vi "capex relay.vi"() -> ()   [LabVIEW 2013]
panel:
  in  "stop":bool
  in  "Relay 4":bool
  in  "Relay 3":bool
  in  "Relay 2":bool
  in  "Relay 1":bool
  # "Relays"
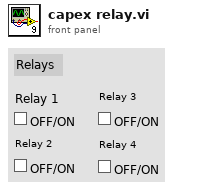
[diagram p1: front panel]
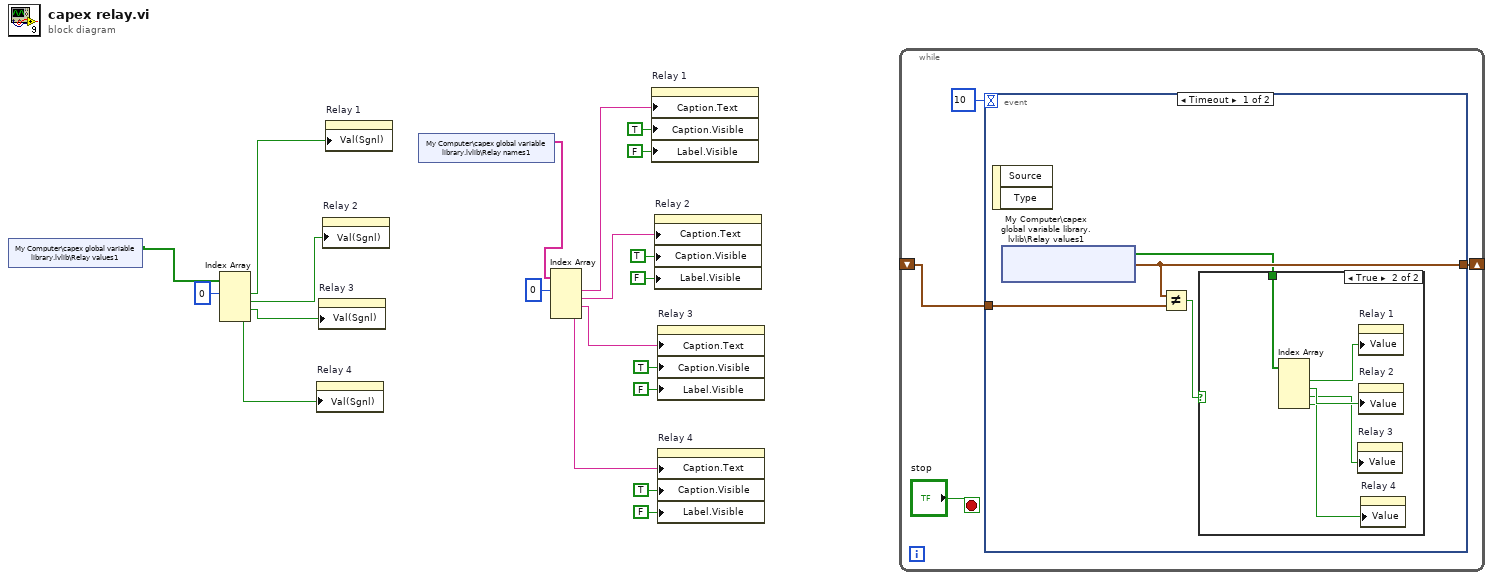
[diagram p0: block diagram]
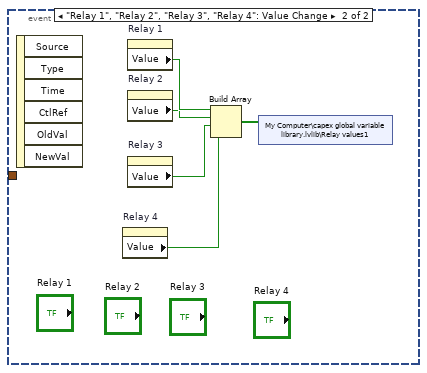
[diagram p3: hidden frame]
diagram:
  n1 = shared-variable "My Computer\\capex global variable library.lvlib\\Relay values1"() -> (w2:bool[])  [unwired: 1 in, 1 out]
  n2 = Index Array(array=w2, index #1=0 ("index")) -> (element #1=w4:bool, element #2=w5:bool, element #3=w6:bool, element #4=w7:bool)  [unwired: 3 in]
  n3 = property on="Relay 4" class="Bool (strict)"("Val(Sgnl)"=w7) -> ()  [unwired: 2 in, 2 out]
  n4 = property on="Relay 3" class="Bool (strict)"("Val(Sgnl)"=w6) -> ()  [unwired: 2 in, 2 out]
  n5 = property on="Relay 2" class="Bool (strict)"("Val(Sgnl)"=w5) -> ()  [unwired: 2 in, 2 out]
  n6 = property on="Relay 1" class="Bool (strict)"("Val(Sgnl)"=w4) -> ()  [unwired: 2 in, 2 out]
  n7 = shared-variable "My Computer\\capex global variable library.lvlib\\Relay names1"() -> (w1:string[])  [unwired: 1 in, 1 out]
  n8 = Index Array(array=w1, index #1=0 ("index")) -> (element #1=w9:string, element #2=w10:string, element #3=w11:string, element #4=w12:string)  [unwired: 3 in]
  n9 = property on="Relay 1" class="Bool (strict)"("Caption.Text"=w9, "Caption.Visible"=TRUE, "Label.Visible"=FALSE) -> ()  [unwired: 2 in, 2 out]
  n10 = property on="Relay 2" class="Bool (strict)"("Caption.Text"=w10, "Caption.Visible"=TRUE, "Label.Visible"=FALSE) -> ()  [unwired: 2 in, 2 out]
  n11 = property on="Relay 3" class="Bool (strict)"("Caption.Text"=w11, "Caption.Visible"=TRUE, "Label.Visible"=FALSE) -> ()  [unwired: 2 in, 2 out]
  n12 = property on="Relay 4" class="Bool (strict)"("Caption.Text"=w12, "Caption.Visible"=TRUE, "Label.Visible"=FALSE) -> ()  [unwired: 2 in, 2 out]
  n13 = while {
    shift-right: [w22] -> _
    shift-left: _ -> [w21]
    stop <- "stop" stop-if-true
    n14 = event shown="[0] Timeout" {
      selector: _ -> [_ _]
      dyn-events: _ -> [_ _]
      timeout: 10 -> [_ _]
      tunnel: [w27 _] -> w22
      tunnel: w21 -> [w28 _]
      event Timeout {
        n15 = event-data() -> ()  [unwired: 1 in, 2 out]
        n16 = shared-variable "My Computer\\capex global variable library.lvlib\\Relay values1"() -> (w25:bool[], w27:timestamp)  [unwired: 1 in, 1 out]
        n17 = Not Equal?(x=w27, y=w28) -> (x != y?=w26:bool)
        n18 = case shown="True" w26 {
          tunnel: w25 -> [_ w33]
          frame False {
          }
          frame True {
            n19 = Index Array(array=w33) -> (element #1=w32:bool, element #2=w31:bool, element #3=w30:bool, element #4=w29:bool)  [unwired: 4 in]
            n20 = property on="Relay 3" class="Bool (strict)"("Value"=w30) -> ()  [unwired: 2 in, 2 out]
            n21 = property on="Relay 1" class="Bool (strict)"("Value"=w32) -> ()  [unwired: 2 in, 2 out]
            n22 = property on="Relay 2" class="Bool (strict)"("Value"=w31) -> ()  [unwired: 2 in, 2 out]
            n23 = property on="Relay 4" class="Bool (strict)"("Value"=w29) -> ()  [unwired: 2 in, 2 out]
          }
        }
      }
      event "Relay 1", "Relay 2", "Relay 3", "Relay 4": Value Change {
        n24 = event-data() -> ()  [unwired: 1 in, 6 out]
        n25 = property on="Relay 4" class="Bool (strict)"() -> ("Value"=w35:bool)  [unwired: 2 in, 2 out]
        n26 = property on="Relay 1" class="Bool (strict)"() -> ("Value"=w38:bool)  [unwired: 2 in, 2 out]
        n27 = property on="Relay 2" class="Bool (strict)"() -> ("Value"=w37:bool)  [unwired: 2 in, 2 out]
        n28 = property on="Relay 3" class="Bool (strict)"() -> ("Value"=w36:bool)  [unwired: 2 in, 2 out]
        n29 = Build Array(w38, w37, w36, w35) -> (w34:bool[])
        n30 = shared-variable "My Computer\\capex global variable library.lvlib\\Relay values1"(w34) -> ()  [unwired: 1 in, 1 out]
      }
    }
  }
